vi "查询启动项.vi"(8 "error in (no error)":errorcluster caption="错误输入（无错误）", 11 "启动文件路径":path) -> (0 "error out":errorcluster caption="错误输出", 3 "包含启动项":bool)   [LabVIEW 2016, in "数据传输系统-05.lvlib"]
uses:
  <vilib>/registry/registry.llb/Registry RtKey.ctl
  <vilib>/registry/registry.llb/Read Registry Value Simple STR.vi
panel:
  out "String/Binary data":string caption="字符串/二进制数据"
  out "values":string[](array[string]) caption="值"
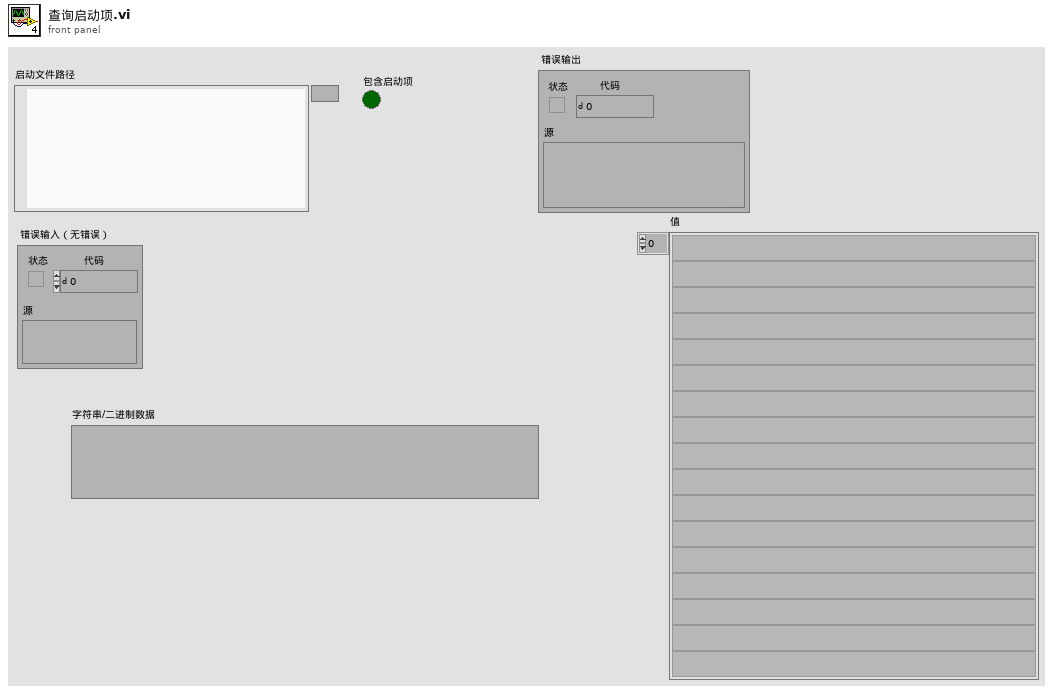
[diagram p1: front panel]
types:
  T1 = typedef "Registry RtKey.ctl" = enum32{"HKEY_CLASSES_ROOT", "HKEY_CURRENT_USER", "HKEY_LOCAL_MACHINE", "HKEY_USERS", "HKEY_PERFORMANCE_DATA", "HKEY_CURRENT_CONFIG", "HKEY_DYN_DATA"}
  T2 = typedef "Registry refnum.ctl" = refnum<k1>
  T3 = cluster{"numValues":i32, "maxValueNameLen":i32, "maxValueDataLen":i32}
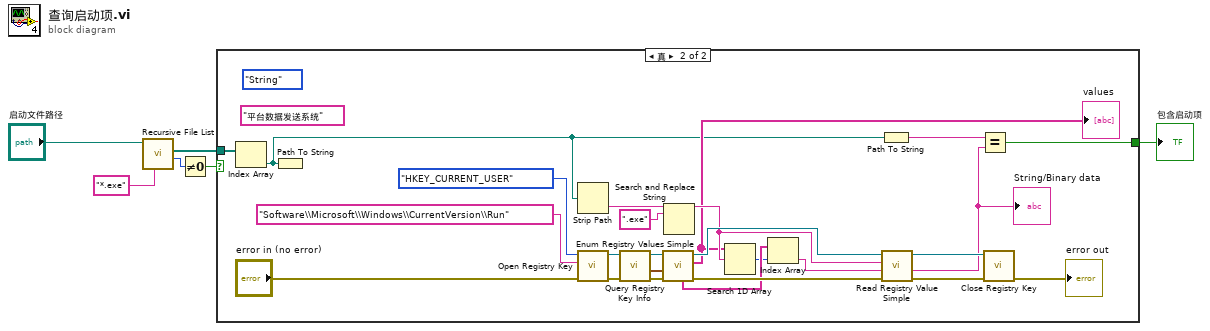
[diagram p0: block diagram]
diagram:
  n1 = call <vilib>:"Recursive File List.vi"("pattern"="*.exe", "Folder Path"="启动文件路径") -> ("Number of Files"=w4:i32, "All Files in Dir"=w5:path[])  [unwired: 5 in, 3 out]
  n2 = Not Equal To 0?(x=w4) -> (x != 0?=w3:bool)
  n3 = case shown="真" w3 {
    tunnel: w5 -> [_ w31]
    tunnel: [_ w10] -> w2
    frame False {
    }
    frame True {
      (unwired) "平台数据发送系统"
      (unwired) enum16{"String", "Binary", "DWORD"}."String" ("simple data type")
      n4 = Index Array(array=w31) -> (element=w9:path)  [unwired: 1 in]
      n5 = Path To String(path=w9) -> ()  [unwired: 1 out]
      n6 = Strip Path(path=w9) -> (name=w30:string)  [unwired: 1 out]
      n7 = call <vilib>:"Open Registry Key.vi"("error in (no error)"="error in (no error)", "subkey"="Software\\Microsoft\\Windows\\CurrentVersion\\Run", "root key (HKEY_LOCAL_MACHINE)"=Registry_RtKey."HKEY_CURRENT_USER") -> ("error out"=w25:errorcluster, "refnum out"=w26:T2)  [unwired: 7 in]
      n8 = call <vilib>:"Query Registry Key Info.vi"("error in (no error)"=w25, "refnum"=w26) -> ("error out"=w20:errorcluster, "value info"=w24:T3, "refnum out"=w21:T2)  [unwired: 5 in, 2 out]
      n9 = call <vilib>:"Enum Registry Values Simple.vi"("error in (no error)"=w20, "value info"=w24, "refnum"=w21) -> ("error out"=w17:errorcluster, "values"=w14:string[], "refnum out"=w19:T2, "String/Binary data"=w13:string[])  [unwired: 3 in, 2 out]
      "values" <- w14
      n10 = Search and Replace String(input string=w30, search string=".exe" ("搜索字符串")) -> (result string=w15:string)  [unwired: 6 in, 3 out]
      n11 = Search 1D Array(1D array=w14, element=w15) -> (index of element=w11:i32)  [unwired: 1 in]
      n12 = Index Array(array=w13, index=w11) -> (element=w12:string)
      n13 = Path To String(path=w9) -> (string=w8:string)
      n14 = call-poly <vilib>:"Read Registry Value Simple.vi"("error in (no error)"=w17, "default data"=w12, "value"=w15, "refnum"=w19) -> ("error out"=w16:errorcluster, "String/Binary data"=w7:string, "refnum out"=w18:T2)  [unwired: 2 in, 1 out]
      "String/Binary data" <- w7
      n15 = Equal?(x=w8, y=w7) -> (x = y?=w10:bool)
      n16 = call <vilib>:"Close Registry Key.vi"("error in (no error)"=w16, "refnum"=w18) -> ("error out"=→"error out":errorcluster)  [unwired: 5 in]
    }
  }
  "包含启动项" <- w2
